vi "Calc_Stats(SubSet).vi"(11 "Image Out":sgl[][](array[numeric])) -> (1 "standard deviation":sgl=0.36516425, 2 "variance":sgl=0.13334493, 3 "mean":sgl=0.551186)   [LabVIEW 2024]
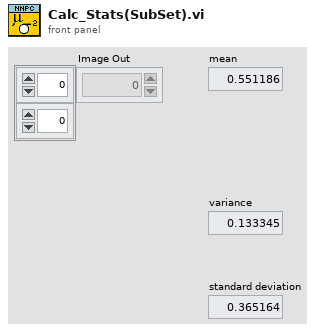
[diagram p1: front panel]
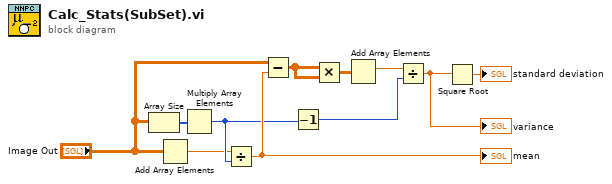
[diagram p0: block diagram]
diagram:
  n1 = Array Size(array="Image Out") -> (size(s)=w4:i32[])
  n2 = Add Array Elements(numeric array="Image Out") -> (sum=w3:sgl)
  n3 = Multiply Array Elements(1:w4) -> (0:w9:i32)
  n4 = Divide(x=w3, y=w9) -> (x/y=w11:sgl)
  "mean" <- w11
  n5 = Subtract(x="Image Out", y=w11) -> (x-y=w5:sgl[][])
  n6 = Decrement(x=w9) -> (x-1=w8:i32)
  n7 = Multiply(x=w5, y=w5) -> (x*y=w6:sgl[][])
  n8 = Add Array Elements(numeric array=w6) -> (sum=w7:sgl)
  n9 = Divide(x=w7, y=w8) -> (x/y=w1:sgl)
  "variance" <- w1
  n10 = Square Root(x=w1) -> (sqrt(x)=→"standard deviation":sgl)
